vi "Sequence.CreateLocalVariables.vi"(8 "error in (no error)":errorcluster, 10 "Steps":T1[](array[typedef]), 11 "Sequence Ref":refnum<k24>) -> (0 "error out":errorcluster, 3 "Sequence Ref out":refnum<k24>)   [LabVIEW 2015, in "Single Station Execution.lvlib"]
uses:
  Single Station Execution.lvlib
  Main.Constants.vi
  NationalInstruments.VeriStand.RealTimeSequenceDefinitionApi
  Types/Step.Types.ctl
  Types/Channel.Properties.ctl
  Types/Compiled.StepElementProperties.ctl
  Types/Compiled.IOStateProperties.ctl
  Types/Conditions.OperationTypes.ctl
  Types/Compiled.StepCondition.ctl
  Types/Compiled.StepProperties.ctl
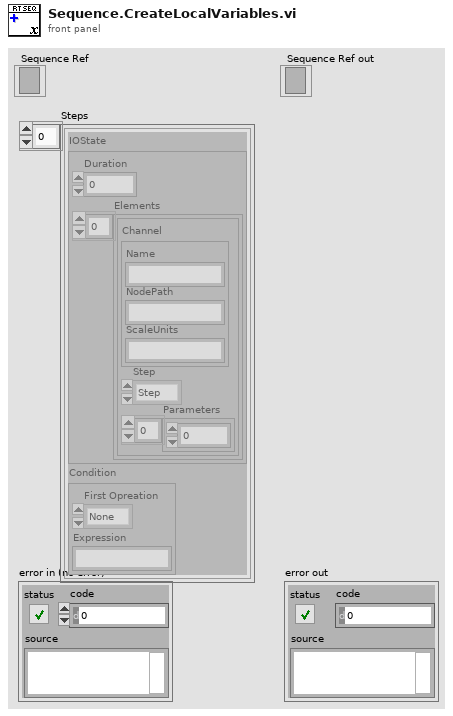
[diagram p1: front panel]
types:
  T1 = typedef "Single Station Execution.lvlib/Compiled.StepProperties.ctl" = cluster{"IOState":T2, "Condition":T6}
  T2 = typedef "Single Station Execution.lvlib/Compiled.IOStateProperties.ctl" = cluster{"Duration":dbl, "Elements":T3[]}
  T3 = typedef "Single Station Execution.lvlib/Compiled.StepElementProperties.ctl" = cluster{"Channel":T4, "Step":T5, "Parameters":dbl[]}
  T4 = typedef "Single Station Execution.lvlib/Channel.Properties.ctl" = cluster{"Name":string, "NodePath":string, "ScaleUnits":string}
  T5 = typedef "Single Station Execution.lvlib/Step.Types.ctl" = enum8{"Step", "iStep", "Ramp", "Unchanged", "Unknown", "Sine", "LogSine", "LinearSine", "ForcedRamp", "Waveform"}
  T6 = typedef "Single Station Execution.lvlib/Compiled.StepCondition.ctl" = cluster{"First Opreation":T7, "Expression":string}
  T7 = typedef "Single Station Execution.lvlib/Conditions.OperationTypes.ctl" = enum8{"None", "&&", "||"}
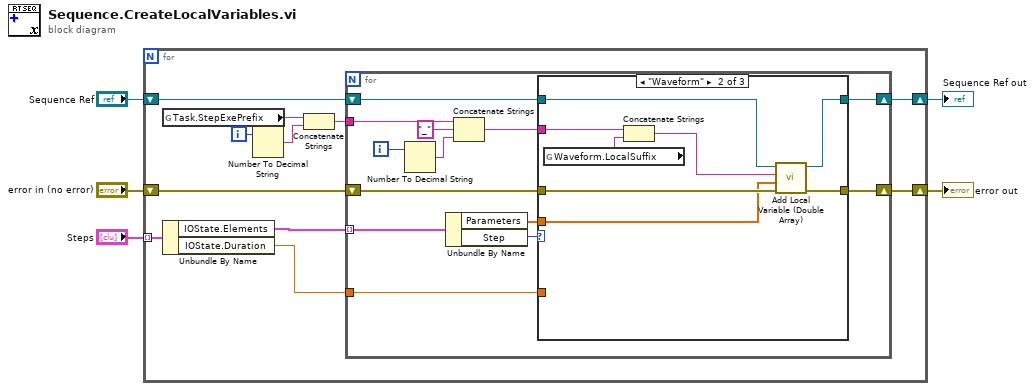
[diagram p0: block diagram]
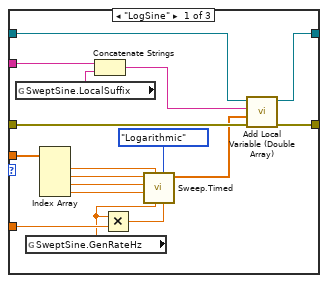
[diagram p2: hidden frame]
diagram:
  n1 = for {
    tunnel: "Steps" -> [w16] mode=indexing
    shift-right: [w11] -> w3
    shift-left: "error in (no error)" -> [w12]
    shift-right: [w13] -> w5
    shift-left: "Sequence Ref" -> [w14]
    i -> [w10]
    n2 = global read "Main.Constants.vi" "Task.StepExePrefix"() -> (w9:string)
    n3 = Unbundle By Name(w16) -> ("IOState.Elements"=w15:T3[], "IOState.Duration"=w6:dbl)
    n4 = Number To Decimal String(number=w10) -> (decimal integer string=w8:string)  [unwired: 1 in]
    n5 = Concatenate Strings(w9, w8) -> (w7:string)
    n6 = for {
      tunnel: w15 -> [w29] mode=indexing
      shift-right: [w23] -> w13
      shift-left: w14 -> [w24]
      shift-right: [w22] -> w11
      shift-left: w12 -> [w28]
      tunnel: w6 -> [w26]
      tunnel: w7 -> [w18]
      i -> [w19]
      n7 = Number To Decimal String(number=w19) -> (decimal integer string=w21:string)  [unwired: 1 in]
      n8 = Unbundle By Name(w29) -> ("Parameters"=w27:dbl[], "Step"=w25:T5)
      n9 = Concatenate Strings(w18, "_" ("string"), w21) -> (w17:string)
      n10 = case shown="\"Waveform\"" w25 {
        tunnel: w28 -> [w44 w54 w55]
        tunnel: w27 -> [w46 w47 _]
        tunnel: w26 -> [w45 _ _]
        tunnel: w24 -> [w43 w53 w56]
        tunnel: [w42 w52 w56] -> w23
        tunnel: [w41 w51 w55] -> w22
        tunnel: w17 -> [w38 w50 _]
        frame "LogSine" {
          n11 = global read "Main.Constants.vi" "SweptSine.LocalSuffix"() -> (w37:string)
          n12 = global read "Main.Constants.vi" "SweptSine.GenRateHz"() -> (w39:dbl)
          n13 = Index Array(array=w46) -> (element #1=w34:dbl, element #2=w35:dbl, element #3=w33:dbl, element #4=w32:dbl)  [unwired: 4 in]
          n14 = Concatenate Strings(w38, w37) -> (w36:string)
          n15 = Multiply(x=w39, y=w45) -> (x*y=w31:dbl)
          n16 = call "Sweep.Timed.vi"("DataPoints"=w31, "frequency spacing"=enum16{"Linear", "Logarithmic"}."Logarithmic", "Fsample (S/s)"=w39, "Offset"=w34, "EndHz"=w32, "StartHz"=w33, "Amplitude"=w35) -> ("Chirp Data"=w40:dbl[])  [unwired: 3 in, 1 out]
          n17 = call "Add Local Variable (Double Array).vi"("error in (no error)"=w44, "Array"=w40, "Identifier"=w36, "Sequence Ref in"=w43) -> ("error out"=w41:errorcluster, "Sequence Ref out"=w42:refnum<k24>)  [unwired: 6 in]
        }
        frame "Waveform" {
          n18 = global read "Main.Constants.vi" "Waveform.LocalSuffix"() -> (w49:string)
          n19 = Concatenate Strings(w50, w49) -> (w48:string)
          n20 = call "Add Local Variable (Double Array).vi"("error in (no error)"=w54, "Array"=w47, "Identifier"=w48, "Sequence Ref in"=w53) -> ("error out"=w51:errorcluster, "Sequence Ref out"=w52:refnum<k24>)  [unwired: 6 in]
        }
        frame Default {
        }
      }
    }
  }
  "Sequence Ref out" <- w5
  "error out" <- w3
